vi "Parse Rx Data.vi"(6 "Trigger":T3, 7 "Scale":T1, 8 "Plot Info":cluster{"Lead":T2, "Filter":bool}[](array[cluster]), 11 "Input Data":i16[](array[numeric])) -> (0 "Pressures":i16[][](array[numeric]), 1 "Gradients":i16[][](array[numeric]), 3 "ECG Data":i16[][](array[numeric]), 4 "Trigger":i16[][](array[numeric]))   [LabVIEW 2016, in "MyHostCode.lvlib"]
uses:
  MyHostCode.lvlib
  Trigger Params.ctl
  FPGACode/Channel Enum.ctl
  FPGACode/Lead Enum.ctl
  <vilib>/Utility/miscctls.llb/LVOffsetAndMultiplierTypeDef.ctl
panel:
  out "Waveform Chart":i16[][](graph)
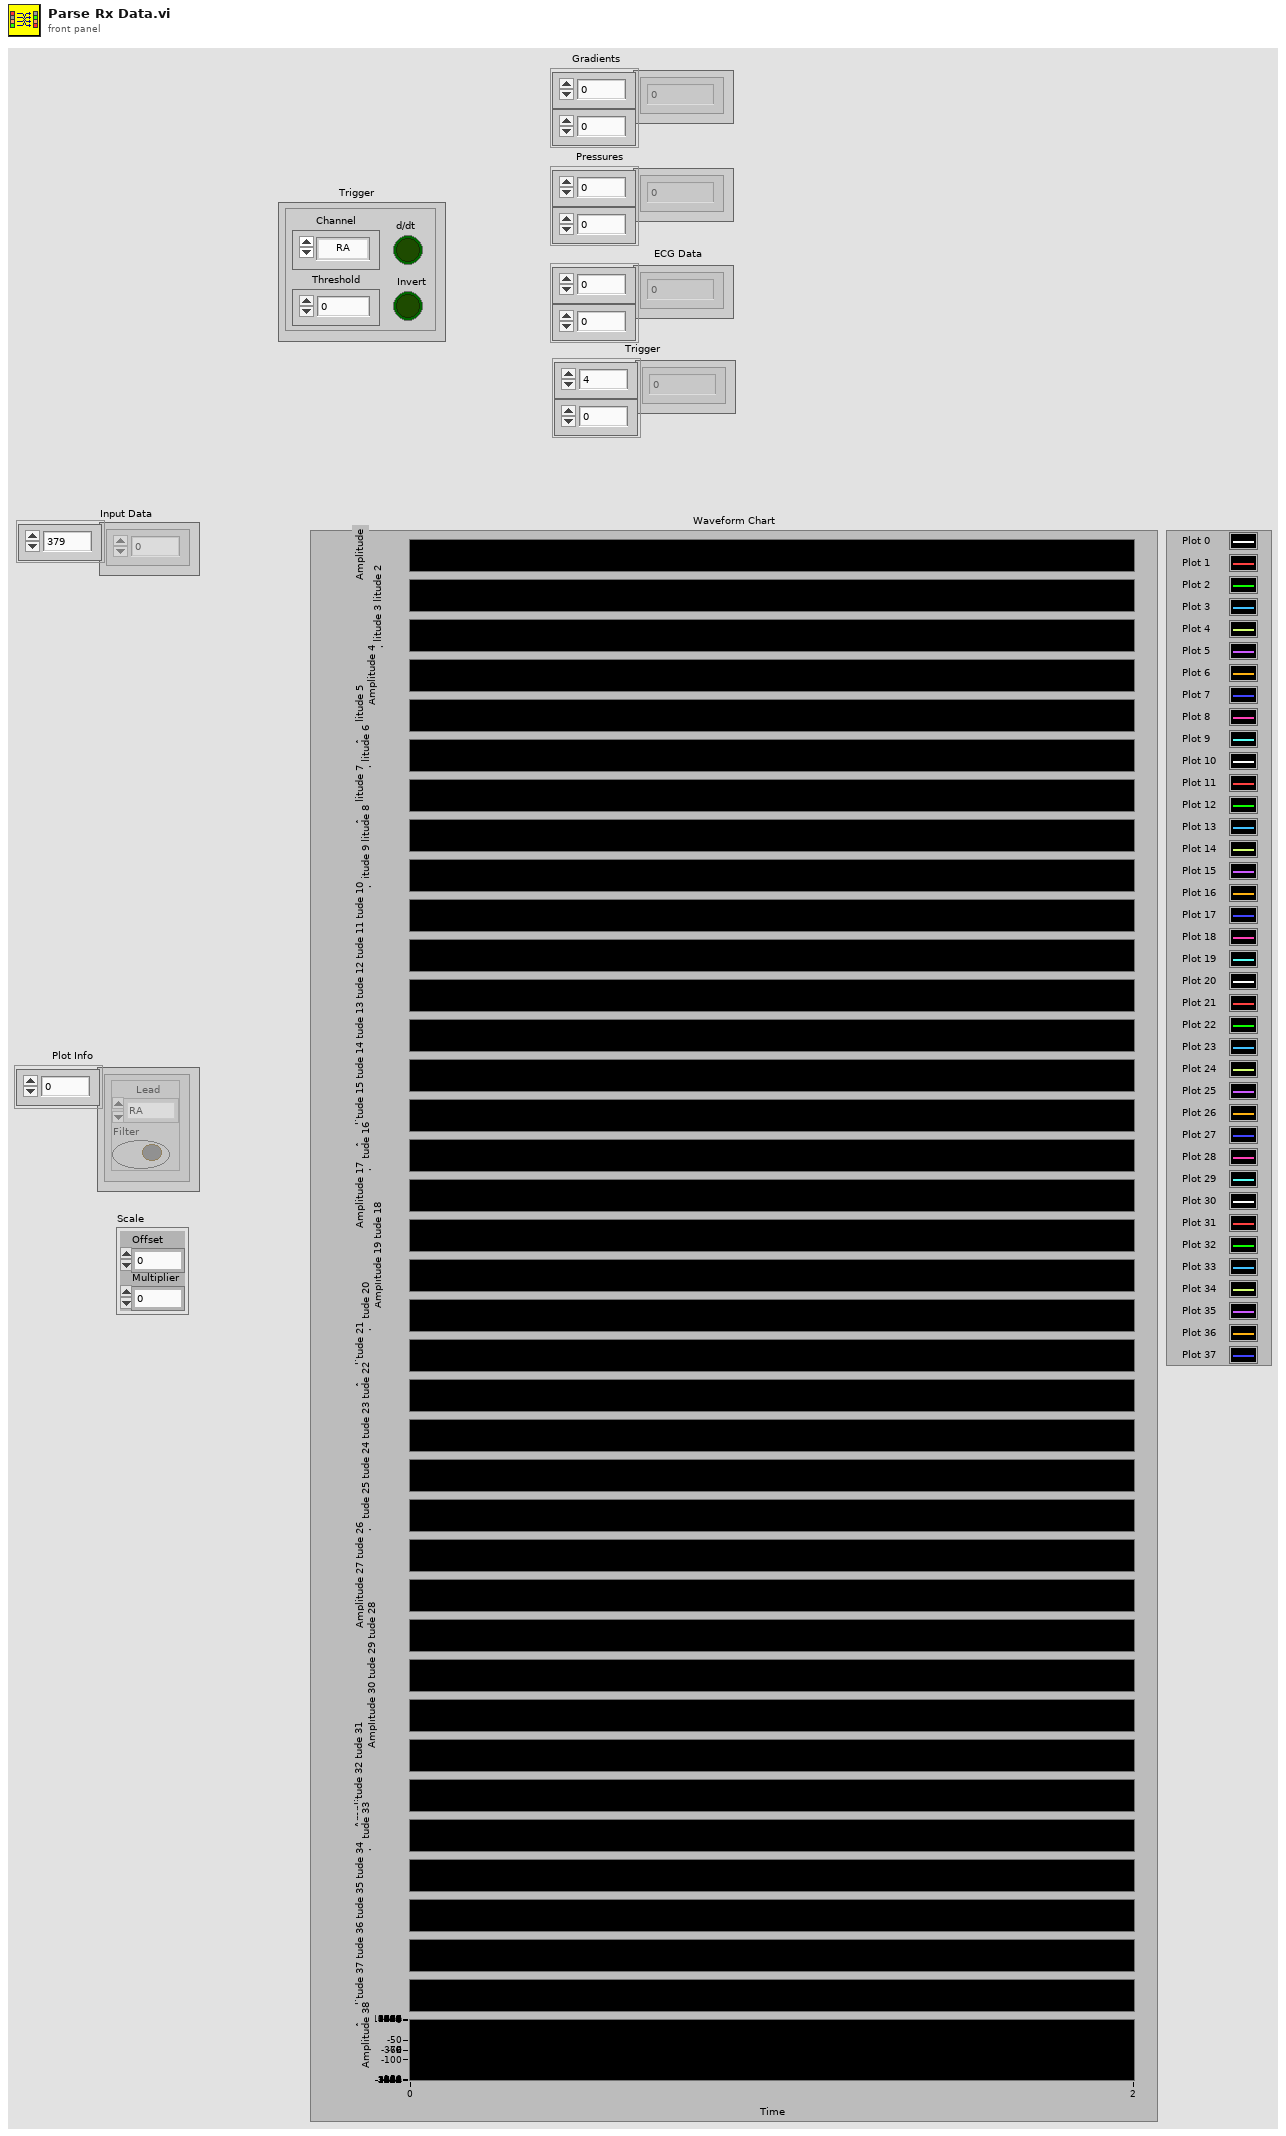
[diagram p1: front panel]
types:
  T1 = typedef "LVOffsetAndMultiplierTypeDef.ctl" = cluster{"Offset":dbl, "Multiplier":dbl}
  T2 = typedef "Lead Enum.ctl" = enum16{"RA", "LA", "LL", "V1", "V2", "V3", "V4", "V5", "V6", "I", "II", "III", "aVR", "aVL", "aVF", "Vw"}
  T3 = typedef "Trigger Params.ctl" = cluster{"Channel":T4, "Threshold":i16, "d/dt":bool, "Invert":bool}
  T4 = typedef "Channel Enum.ctl" = enum16{"RA", "LA", "LL", "V1", "V2", "V3", "V4", "V5", "V6", "I", "II", "III", "aVR", "aVL", "aVF", "Vw", "IBP1", "IBP2"}
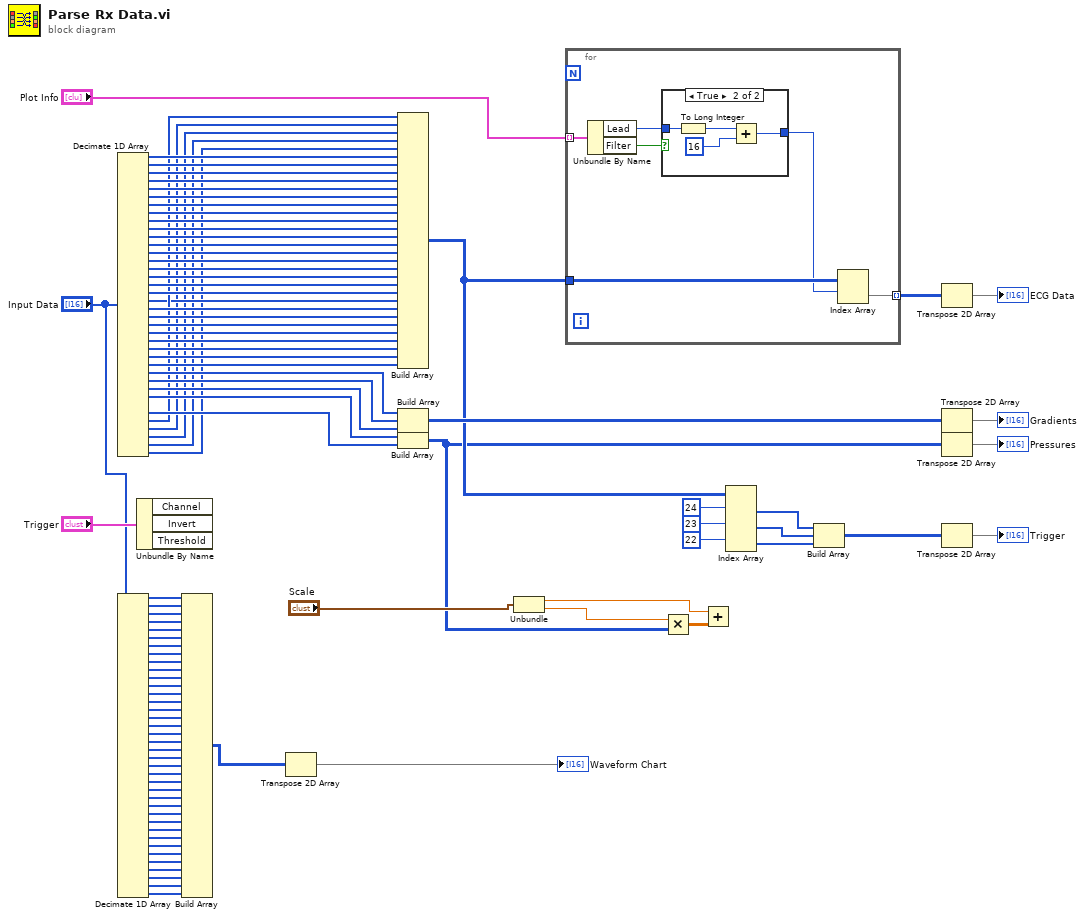
[diagram p0: block diagram]
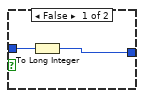
[diagram p2: hidden frame]
diagram:
  n1 = Decimate 1D Array("Input Data") -> (w99:i16[], w98:i16[], w97:i16[], w96:i16[], w95:i16[], w94:i16[], w93:i16[], w92:i16[], w91:i16[], w90:i16[], w89:i16[], w88:i16[], w87:i16[], w86:i16[], w85:i16[], w84:i16[], w83:i16[], w82:i16[], w21:i16[], w81:i16[], w80:i16[], w79:i16[], w78:i16[], w77:i16[], w76:i16[], w75:i16[], w74:i16[], w23:i16[], w24:i16[], w25:i16[], w26:i16[], w27:i16[], w22:i16[], w20:i16[], w19:i16[], w18:i16[], w17:i16[])  [unwired: 1 out]
  n2 = Decimate 1D Array("Input Data") -> (w36:i16[], w37:i16[], w38:i16[], w39:i16[], w40:i16[], w41:i16[], w42:i16[], w43:i16[], w44:i16[], w45:i16[], w46:i16[], w47:i16[], w48:i16[], w49:i16[], w50:i16[], w51:i16[], w52:i16[], w53:i16[], w54:i16[], w55:i16[], w56:i16[], w57:i16[], w58:i16[], w59:i16[], w60:i16[], w61:i16[], w62:i16[], w63:i16[], w64:i16[], w65:i16[], w66:i16[], w67:i16[], w34:i16[], w33:i16[], w32:i16[], w31:i16[], w30:i16[], w29:i16[])
  n3 = Unbundle By Name("Trigger") -> ()  [unwired: 3 out]
  n4 = Build Array(w36, w37, w38, w39, w40, w41, w42, w43, w44, w45, w46, w47, w48, w49, w50, w51, w52, w53, w54, w55, w56, w57, w58, w59, w60, w61, w62, w63, w64, w65, w66, w67, w34, w33, w32, w31, w30, w29) -> (w28:i16[][])
  n5 = Transpose 2D Array(2D array=w28) -> (transposed array=→"Waveform Chart":i16[][])
  n6 = Build Array(w22, w20, w19, w18, w17, w99, w98, w97, w96, w95, w94, w93, w92, w91, w90, w89, w88, w87, w86, w85, w84, w83, w82, w21, w81, w80, w79, w78, w77, w76, w75, w74) -> (w11:i16[][])
  n7 = Build Array(w23, w24, w25) -> (w73:i16[][])
  n8 = Build Array(w26, w27) -> (w7:i16[][])
  n9 = Unbundle("Scale") -> ("Offset"=w13:dbl, "Multiplier"=w15:dbl)
  n10 = for {
    tunnel: w11 -> [w101]
    tunnel: "Plot Info" -> [w105] mode=indexing
    tunnel: [w102] -> w70 mode=indexing
    n11 = Unbundle By Name(w105) -> ("Lead"=w103:T2, "Filter"=w104:bool)
    n12 = case shown="True" w104 {
      tunnel: w103 -> [w107 w111]
      tunnel: [w106 w108] -> w100
      frame False {
        n13 = To Long Integer(number=w107) -> (32bit integer=w106:i32)
      }
      frame True {
        n14 = To Long Integer(number=w111) -> (32bit integer=w109:i32)
        n15 = Add(x=w109, y=16) -> (x+y=w108:i32)
      }
    }
    n16 = Index Array(array=w101, index (row)=w100) -> (element=w102:i16[])  [unwired: 1 in]
  }
  n17 = Multiply(x=w15, y=w7) -> (x*y=w14:dbl[][])
  n18 = Add(x=w13, y=w14) -> ()  [unwired: 1 out]
  n19 = Index Array(array=w11, index (row) #1=24 ("index (row)"), index (row) #2=23 ("index (row)"), index (row) #3=22 ("index (row)")) -> (element #1=w5:i16[], element #2=w3:i16[], element #3=w1:i16[])  [unwired: 3 in]
  n20 = Build Array(w5, w3, w1) -> (w10:i16[][])
  n21 = Transpose 2D Array(2D array=w70) -> (transposed array=→"ECG Data":i16[][])
  n22 = Transpose 2D Array(2D array=w73) -> (transposed array=→"Gradients":i16[][])
  n23 = Transpose 2D Array(2D array=w7) -> (transposed array=→"Pressures":i16[][])
  n24 = Transpose 2D Array(2D array=w10) -> (transposed array=→"Trigger":i16[][])
